vi "Generate Saw.vi"(2 "V in y":dbl, 3 "V in x":dbl, 4 "VNT'y":dbl, 5 "VNT'x":dbl) -> (0 "V out y":dbl[](array[numeric]), 1 "V out x":dbl[](array[numeric]))   [LabVIEW 2013]
uses:
  <vilib>/measure/NI_MABase.lvlib
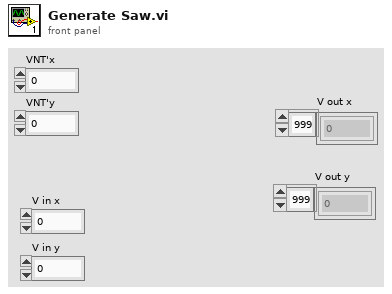
[diagram p1: front panel]
types:
  T1 = enum16{"Sine Wave", "Triangle Wave", "Square Wave", "Sawtooth Wave"}
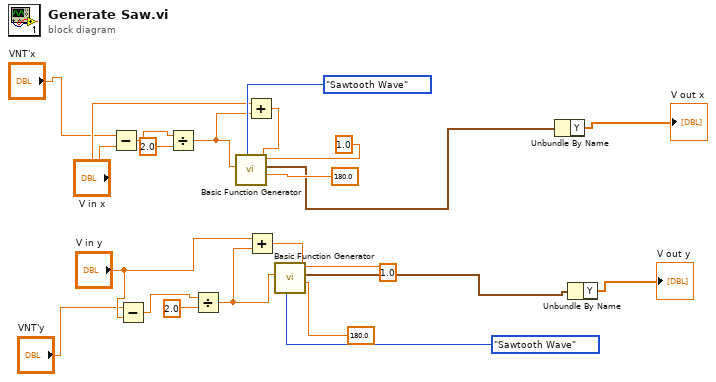
[diagram p0: block diagram]
diagram:
  n1 = Subtract(x="VNT'x", y="V in x") -> (x-y=w15:dbl)
  n2 = Subtract(x="VNT'y", y="V in y") -> (x-y=w10:dbl)
  n3 = Divide(x=w15, y=2.0) -> (x/y=w13:dbl)
  n4 = Divide(x=w10, y=2.0) -> (x/y=w9:dbl)
  n5 = Add(x="V in x", y=w13) -> (x+y=w12:dbl)
  n6 = call <vilib>:"Basic Function Generator.vi"("offset"=w12, "signal type"=T1."Sawtooth Wave", "phase"=180.0, "amplitude"=w13, "frequency"=1.0) -> ("signal out"=w6:waveform(dbl))  [unwired: 4 in, 2 out]
  n7 = Add(x="V in y", y=w9) -> (x+y=w8:dbl)
  n8 = call <vilib>:"Basic Function Generator.vi"("offset"=w8, "signal type"=T1."Sawtooth Wave", "phase"=180.0, "amplitude"=w9, "frequency"=1.0) -> ("signal out"=w5:waveform(dbl))  [unwired: 4 in, 2 out]
  n9 = Unbundle By Name(w6) -> ("Y"=→"V out x":dbl[])
  n10 = Unbundle By Name(w5) -> ("Y"=→"V out y":dbl[])
